vi "Initialize.vi"(7 "SMO.InstrumentDriver in":refnum<class "SMO.InstrumentDriver.lvclass">, 8 "error in (no error)":errorcluster, 10 "Subsystem Name (optional)":string, 11 "Configuration":variant) -> (0 "error out":errorcluster, 2 "SMO name":string, 3 "SMO.InstrumentDriver out":refnum<class "SMO.InstrumentDriver.lvclass">)   [LabVIEW 2013, in "SMO.InstrumentDriver.lvclass"]
uses:
  SMO.InstrumentDriver.lvclass
  <vilib>/JKI/JKI SMO/SMO/SMO.lvclass
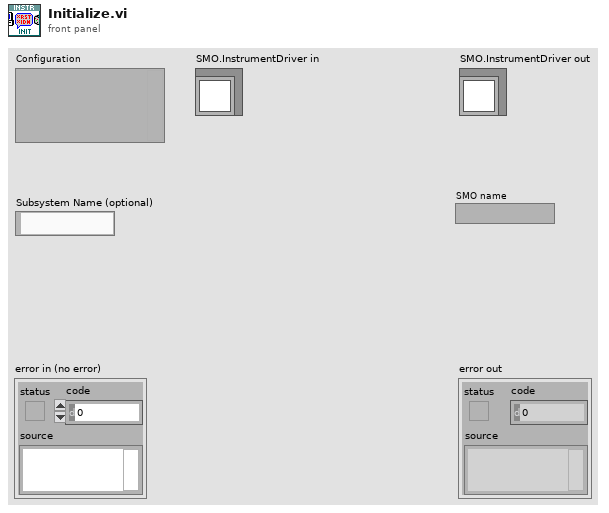
[diagram p1: front panel]
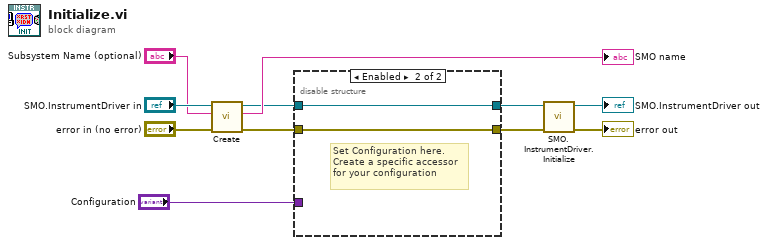
[diagram p0: block diagram]
diagram:
  n1 = call <vilib>:"Create.vi"("error in (no error)"="error in (no error)", "Subsystem Name (optional)"="Subsystem Name (optional)", "SMO"="SMO.InstrumentDriver in") -> ("error out"=w2:errorcluster, "SMO name"=→"SMO name":string, "SMO out"=w5:refnum<class "SMO.InstrumentDriver.lvclass">)  [unwired: 6 in]
  n2 = disable-structure shown="Enabled" {
    disable-tunnel: w5 -> [w13 w15]
    disable-tunnel: [w13 w15] -> w4
    disable-tunnel: [w12 w14] -> w3
    disable-tunnel: w2 -> [w12 w14]
    disable-tunnel: "Configuration" -> [_ _]
    frame Disabled {
    }
    frame Enabled {
      # "Set Configuration here.\nCreate a specific accessor\nfor your configuration"
    }
  }
  n3 = call-dynamic "SMO.InstrumentDriver.Initialize.vi"("error in (no error)"=w3, "SMO.Instrument"=w4) -> ("error out"=→"error out":errorcluster, "SMO.Instrument out"=→"SMO.InstrumentDriver out":refnum<class "SMO.InstrumentDriver.lvclass">)  [unwired: 8 in]
